vi "Config-System.vi"() -> ()   [LabVIEW 2016]
uses:
  <vilib>/Utility/error.llb/DialogType.ctl
  DAQ-Display/PanelSplitToolkit/QueueManager.llb/CreatQueue.vi
  DAQ-Display/PanelSplitToolkit/QueueManager.llb/Remove.vi
  DAQ-Display/PanelSplitToolkit/QueueManager.llb/Destroy.vi
  DAQ-Display/PanelSplitToolkit/QueueManager.llb/Valid?.vi
  DAQ-Display/PanelSplitToolkit/QueueManager.llb/Insert.vi
panel:
  in  "关注参数个数":u8=4 min=4 max=16
  in  "Caller":string caption="文件名："
  in  "手动挑点模板":path
  in  "存储路径":path
  in  "自动挑点注释":string caption="文件名："
  in  "文件存储方式":enum16{"不连续存储", "连续存储"}(ring)=enum."连续存储"
  in  "挑点模式":enum16{"不挑点", "自动挑点", "手动挑点"}(ring)=enum."自动挑点"
  in  "文件名":string caption="文件名："
  in  "默认波形图个数":u8=4 min=1 max=4
  in  "挑点间隔":i32=2
  # "存储设置"
  # "存储方式："
  # "文件夹路径："
  # "默认文件名："
  # "挑点设置"
  # "挑点模式："
  # "自动挑点间隔："
  # "秒"
  # "手动挑点模板："
  # "自动挑点注释："
  # "显示设置"
  # "个"
  # "默认图形窗口 :"
  # "个"
  # "关注参数个数 :"
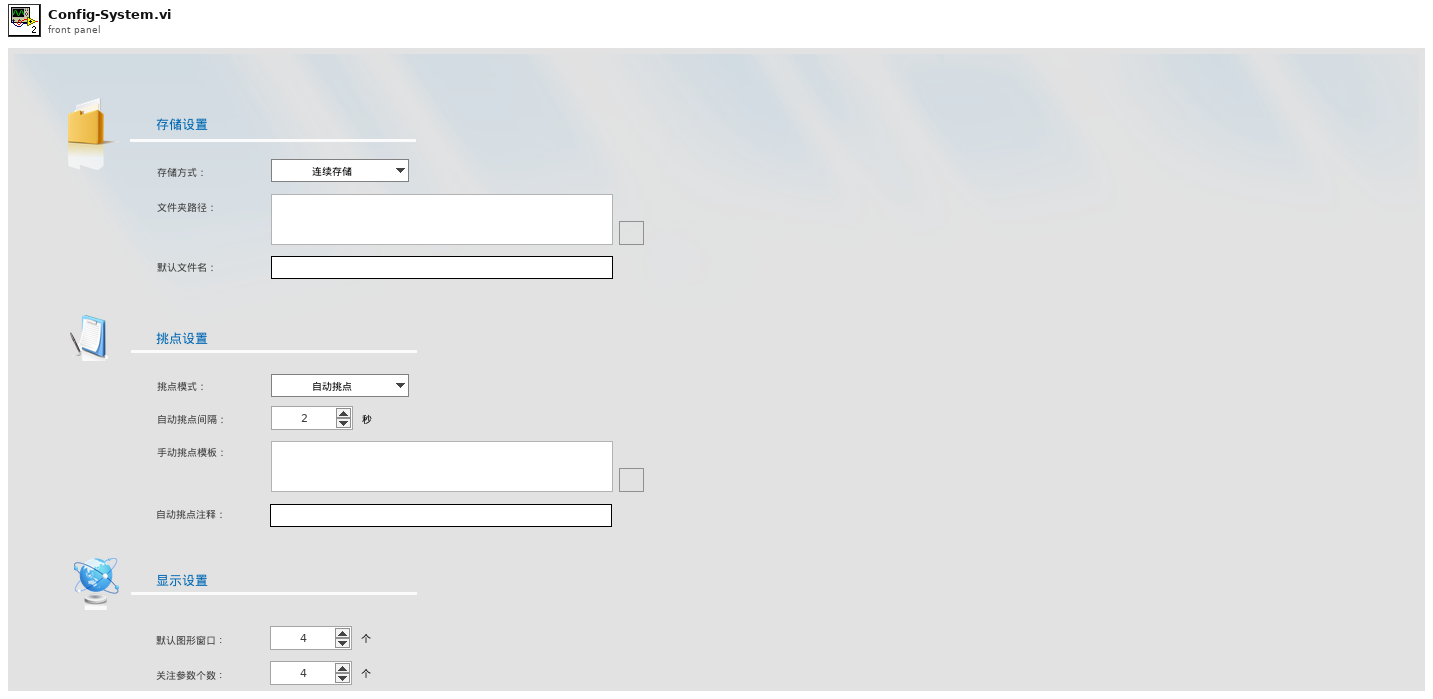
[diagram p1: front panel]
types:
  T1 = cluster{"error":errorcluster, "LocalQ":cluster{"LQName":string, "LQEvent":string, "LQData":variant}, "HighQ":cluster{"HQName":string, "HQEvent":string, "HQData":variant}}
  T2 = enum32{"Invalid", "Standard", "Closed", "Hidden", "Minimized", "Maximized"}
  T3 = typedef "DialogType.ctl" = u16
  T4 = typedef "Global para Config.ctl" = cluster{"连续存储设置":cluster{"Save Mode":i32, "Sel Save Mode":i32, "FolderPath":path, "Filename":string, "Explation":string, "AutoPoint":i32, "Template":path}, "Latest Prj":path, "Tdms Ref*":refnum<k34>, "默认波形图个数":u8, "列表列数":u8}
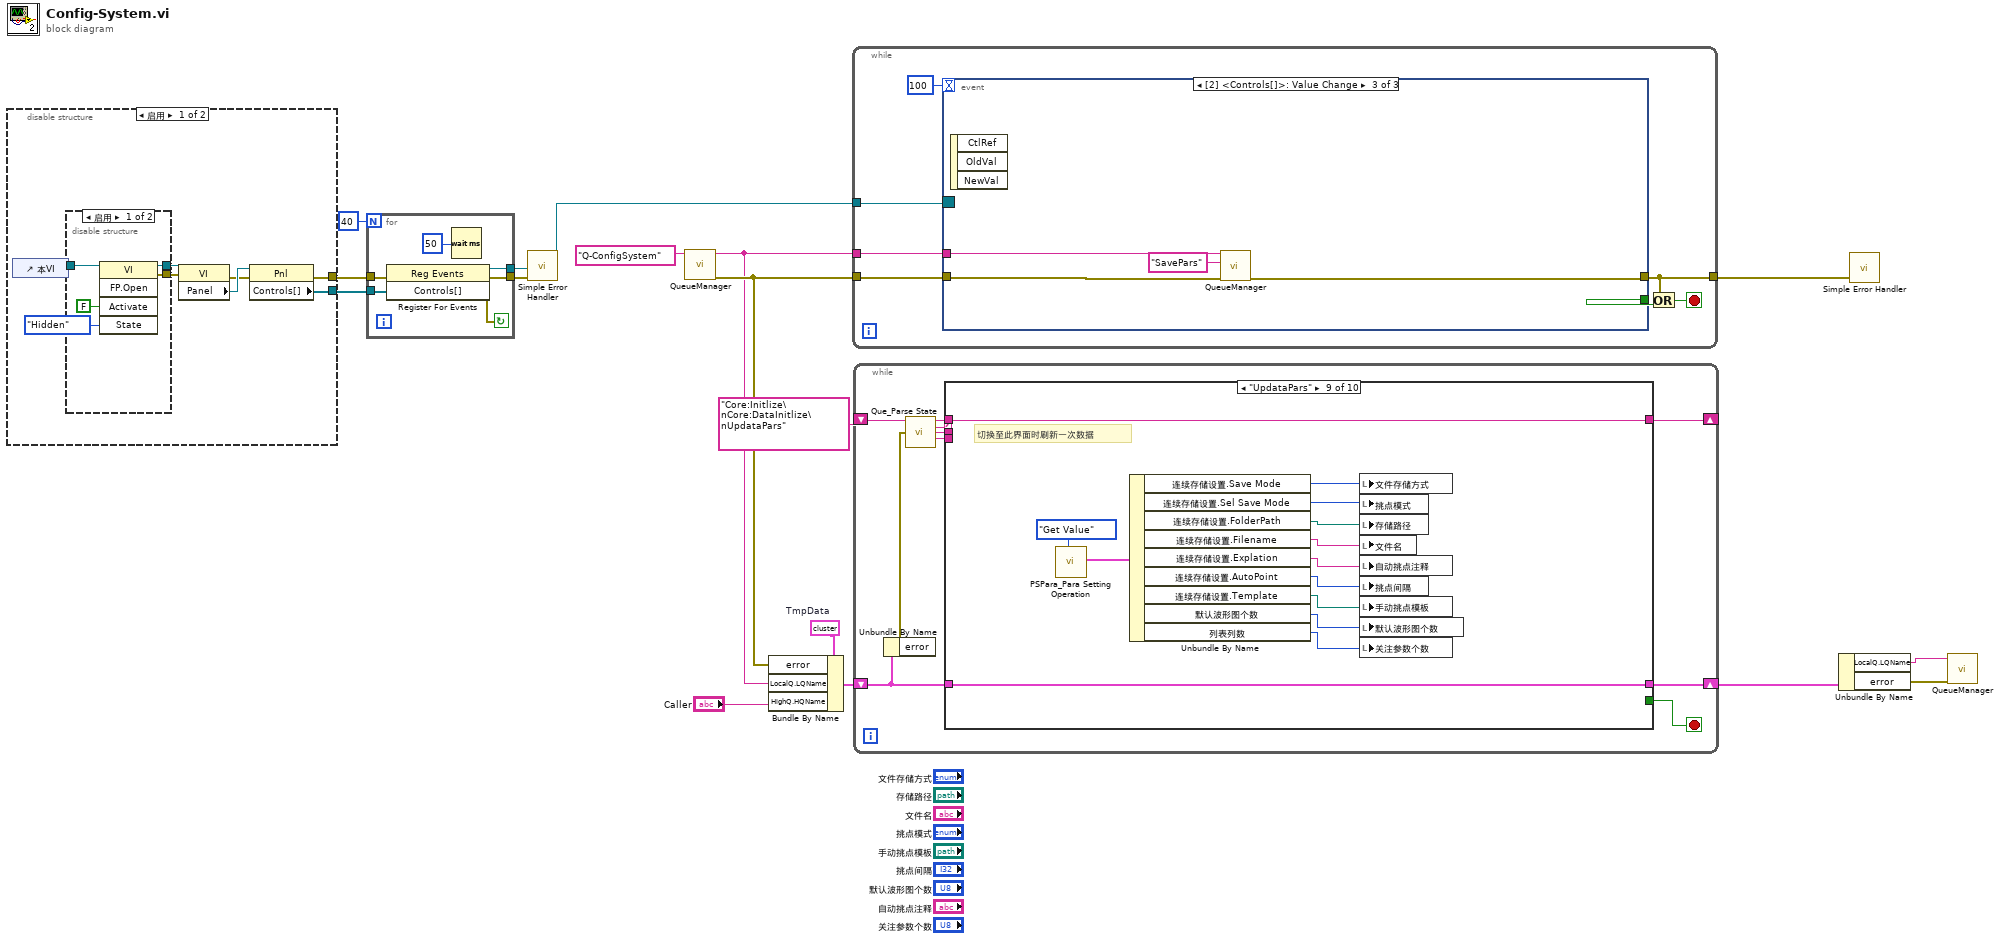
[diagram p0: block diagram]
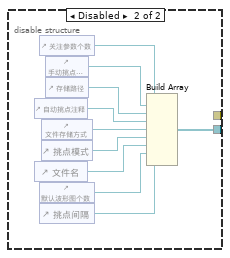
[diagram p3: hidden frame]
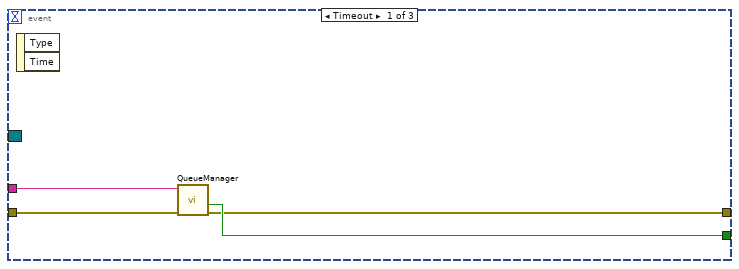
[diagram p4: hidden frame]
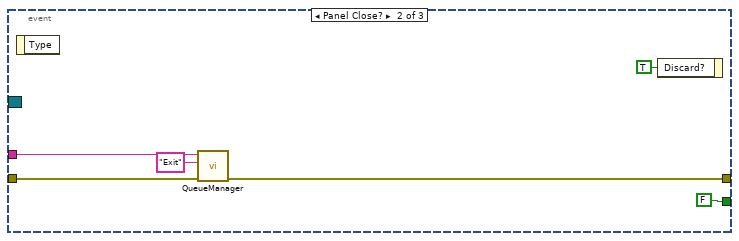
[diagram p5: hidden frame]
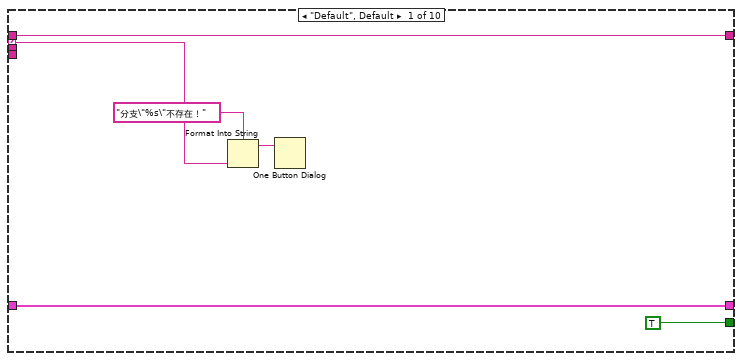
[diagram p6: hidden frame]
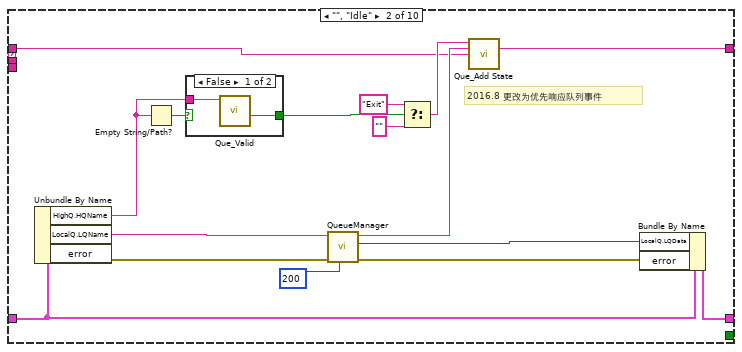
[diagram p7: hidden frame]
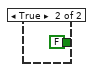
[diagram p8: hidden frame]
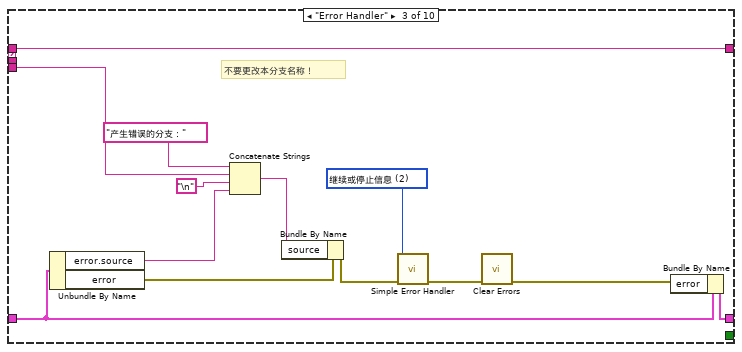
[diagram p9: hidden frame]
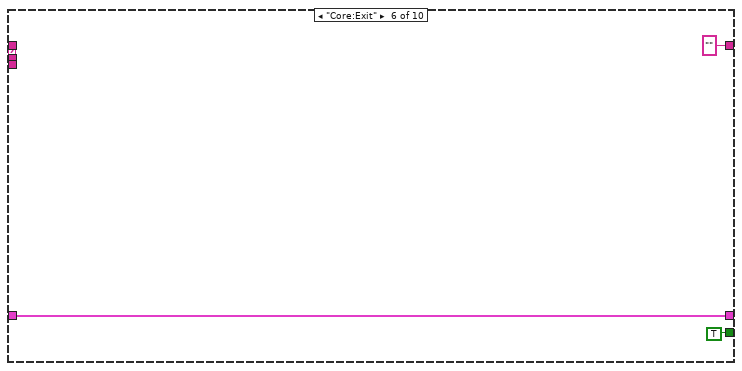
[diagram p12: hidden frame]
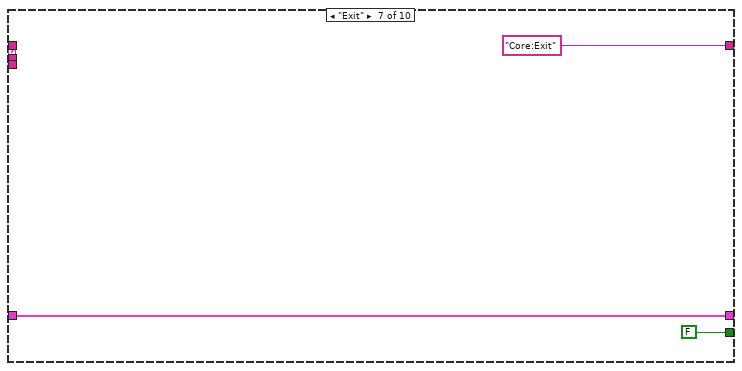
[diagram p13: hidden frame]
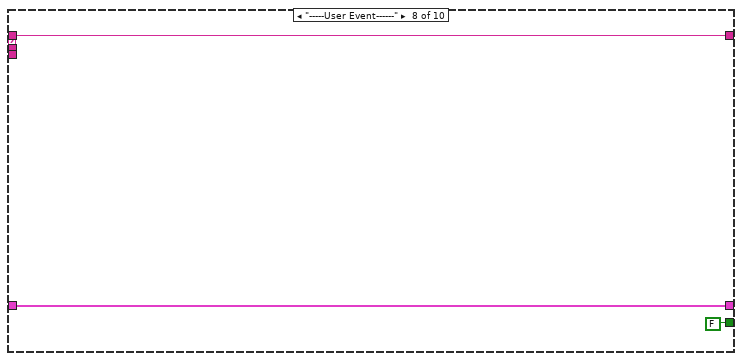
[diagram p14: hidden frame]
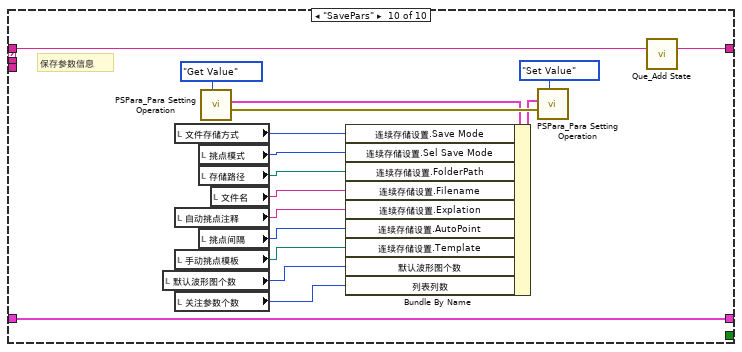
[diagram p15: hidden frame]
diagram:
  w12 = T1 {"error"={"status"=FALSE, "code"=0, "source"=""}, "LocalQ"={"LQName"="", "LQEvent"="", "LQData"=variant}, "HighQ"={"HQName"="", "HQEvent"="", "HQData"=variant}}  # TmpData
  n1 = disable-structure shown="启用" {
    disable-tunnel: [w21 w30] -> w5
    disable-tunnel: [w20 _] -> w4
    frame Enabled {
      n2 = control-ref of="本VI"() -> (w17:refnum<vi>)
      n3 = disable-structure shown="启用" {
        disable-tunnel: [w28 w29] -> w19
        disable-tunnel: [w27 _] -> w18
        disable-tunnel: w17 -> [w26 w29]
        frame Enabled {
          n4 = invoke class="VI" method="FP.Open"(reference=w26, "Activate"=FALSE ("激活？"), "State"=T2."Hidden" ("状态")) -> (reference out=w28:refnum<vi>, error out=w27:errorcluster)  [unwired: 2 in, 3 out]
        }
        frame Disabled {
        }
      }
      n5 = property class="VI"(reference=w19, error in=w18) -> (error out=w22:errorcluster, "Panel"=w23:refnum<vi>)  [unwired: 1 out]
      n6 = property class="Pnl"(reference=w23, error in=w22) -> (error out=w20:errorcluster, "Controls[]"=w21:refnum<vi>[])  [unwired: 1 out]
    }
    frame Disabled {
      n7 = control-ref of="自动挑点注释"() -> (w36:refnum<vi>)
      n8 = control-ref of="文件名"() -> (w33:refnum<vi>)
      n9 = control-ref of="关注参数个数"() -> (w39:refnum<vi>)
      n10 = control-ref of="默认波形图个数"() -> (w32:refnum<vi>)
      n11 = control-ref of="挑点间隔"() -> (w31:refnum<vi>)
      n12 = control-ref of="文件存储方式"() -> (w35:refnum<vi>)
      n13 = control-ref of="挑点模式"() -> (w34:refnum<vi>)
      n14 = control-ref of="手动挑点模板"() -> (w38:refnum<vi>)
      n15 = control-ref of="存储路径"() -> (w37:refnum<vi>)
      n16 = Build Array(w39, w38, w37, w36, w35, w34, w33, w32, w31) -> (w30:refnum<vi>[])
    }
  }
  n17 = for {
    N: 40 -> [_]
    tunnel: w5 -> [w44]
    tunnel: [w42] -> w3
    tunnel: w4 -> [w43]
    tunnel: [w40] -> w1
    stop <- w40 continue-if-true
    n18 = register-events(error in=w43, w44) -> (reference out=w42:refnum<event-registration>, error out=w40:errorcluster)  [unwired: 1 in]
    n19 = Wait (ms)(milliseconds to wait=u32 50 ("等待时间（毫秒）")) -> ()  [unwired: 1 out]
  }
  n20 = call <vilib>:"Simple Error Handler.vi"("error in (no error)"=w1) -> ()  [unwired: 4 in, 5 out]
  n21 = call-poly "QueueManager.vi"("QueueName"="Q-ConfigSystem") -> ("error out"=w8:errorcluster, "QueueName out"=w6:string)  [unwired: 9 in]
  n22 = Bundle By Name(cluster=w12, "error"=w8, "LocalQ.LQName"=w6, "HighQ.HQName"="Caller") -> (w11:T1)
  n23 = while {
    tunnel: w8 -> [w50]
    tunnel: w6 -> [w51]
    tunnel: [w47] -> w13
    tunnel: w3 -> [w45]
    stop <- w48 stop-if-true
    n24 = event shown="[2] <Controls[]>: Value Change" {
      selector: w45 -> [_ _ _]
      dyn-events: _ -> [_ _ _]
      timeout: 100 -> [_ _ _]
      tunnel: [w53 FALSE _] -> w49
      tunnel: w51 -> [w55 w60 w64]
      tunnel: w50 -> [w54 w59 w65]
      tunnel: [w52 w58 w63] -> w47
      event Timeout {
        n25 = event-data() -> ()  [unwired: 1 in, 2 out]
        n26 = call-poly "QueueManager.vi"("error in (no error)"=w54, "Queue Name(unamed)"=w55) -> ("error out"=w52:errorcluster, "Not Exist?"=w53:bool)  [unwired: 8 in]
      }
      event Panel Close? {
        n27 = event-data() -> ()  [unwired: 1 in, 1 out]
        n28 = call-poly "QueueManager.vi"("error in"=w59, "Event"="Exit", "QueueName"=w60) -> ("error out"=w58:errorcluster)  [unwired: 7 in, 1 out]
        n29 = event-data("Discard?"=TRUE ("放弃？")) -> ()  [unwired: 1 in, 1 out]
      }
      event Value Change {
        n30 = event-data() -> ()  [unwired: 1 in, 3 out]
        n31 = call-poly "QueueManager.vi"("error in"=w65, "Event"="SavePars", "QueueName"=w64) -> ("error out"=w63:errorcluster)  [unwired: 7 in, 1 out]
      }
    }
    n32 = Or(x=w47, y=w49) -> (x .or. y?=w48:bool)
  }
  n33 = while {
    shift-right: [w69] -> w14
    shift-left: w11 -> [w70]
    shift-right: [w68] -> _
    shift-left: "Core:Initlize\nCore:DataInitlize\nUpdataPars" -> [w75]
    stop <- w72 stop-if-true
    n34 = Unbundle By Name(w70) -> ("error"=w71:errorcluster)
    n35 = call "Que_Parse State.vi"("State Queue"=w75, "Error In (no error)"=w71) -> ("Remaining States"=w74:string, "Current State"=w73:string, "Arguments"=w67:string, "PreState"=w66:string)  [unwired: 10 in]
    n36 = case shown="\"UpdataPars\"" w73 {
      selector: w73 -> [w79 _ _ _ _ _ _ _ _ _]
      tunnel: w74 -> [w80 w82 w113 w115 w117 _ _ w124 w138 w155]
      tunnel: w67 -> [_ _ _ _ _ _ _ _ _ _]
      tunnel: [TRUE _ _ _ _ TRUE FALSE FALSE _ _] -> w72
      tunnel: w70 -> [w81 w92 w110 w114 w116 w119 w122 w125 w139 w156]
      tunnel: [w81 w96 w109 w114 w116 w119 w122 w125 w139 w156] -> w69
      tunnel: [w80 w94 w113 w115 w117 "" ("Remaining States") "Core:Exit" ("Remaining States") w124 w138 w154] -> w68
      tunnel: w66 -> [_ _ w107 _ _ _ _ _ _ _]
      frame "Default", Default {
        n37 = Format Into String(format string="分支\"%s\"不存在！" ("格式字符串"), w79) -> (resulting string=w78:string)  [unwired: 2 in, 1 out]
        n38 = One Button Dialog(message=w78) -> ()  [unwired: 1 in, 1 out]
      }
      frame "", "Idle" {
        # "2016.8 更改为优先响应队列事件"
        n39 = Unbundle By Name(w92) -> ("HighQ.HQName"=w86:string, "LocalQ.LQName"=w91:string, "error"=w90:errorcluster)
        n40 = Empty String/Path?(string/path=w86) -> (empty?=w89:bool)
        n41 = case shown="False" w89 {
          tunnel: [w99 FALSE ("Not Exist?")] -> w88
          tunnel: w86 -> [w98 _]
          frame False {
            n42 = call "Que_Valid.vi"("Queue Name(unamed)"=w98) -> ("Not Exist?"=w99:bool)  [unwired: 9 in, 1 out]
          }
          frame True {
          }
        }
        n43 = call-poly "QueueManager.vi"("Time out(-1)"=200, "error in (no error)"=w90, "Queue Name"=w91) -> ("error out"=w97:errorcluster, "Data"=w95:variant, "Event"=w83:string)  [unwired: 5 in, 1 out]
        n44 = Select(t="Exit" ("Event"), s=w88, f="") -> (s? t:f=w84:string)
        n45 = call "Que_Add State.vi"("State(s) in Front (\"\")"=w84, "State(s) in (\"\")"=w83, "State(s) at Back (\"\")"=w82) -> ("States Out"=w94:string)  [unwired: 12 in]
        n46 = Bundle By Name(cluster=w92, "LocalQ.LQData"=w95, "error"=w97) -> (w96:T1)
      }
      frame "Error Handler" {
        w108 = T3 2 items=["无对话框", "确定信息", "继续或停止信息", "确定信息＋警告", "继续/停止+警告"] ("type of dialog (OK msg:1)")
        # "不要更改本分支名称！"
        n47 = Unbundle By Name(w110) -> ("error.source"=w101:string, "error"=w103:errorcluster)
        n48 = Concatenate Strings("产生错误的分支：" ("字符串"), w107, "\n", w101) -> (w104:string)
        n49 = Bundle By Name(cluster=w103, "source"=w104) -> (w102:errorcluster)
        n50 = call <vilib>:"Simple Error Handler.vi"("type of dialog (OK msg:1)"=w108, "error in (no error)"=w102) -> ("error out"=w111:errorcluster)  [unwired: 3 in, 4 out]
        n51 = call <vilib>:"Clear Errors.vi"("error in (no error)"=w111) -> ("error out"=w112:errorcluster)  [unwired: 5 in, 1 out]
        n52 = Bundle By Name(cluster=w110, "error"=w112) -> (w109:T1)
      }
      frame "Core:Initlize" {
      }
      frame "Core:DataInitlize" {
      }
      frame "Core:Exit" {
      }
      frame "Exit" {
      }
      frame "-----User Event------" {
      }
      frame "UpdataPars" {
        # "切换至此界面时刷新一次数据"
        n53 = call "PSPara_Para Setting Operation.vi"("Operation"=enum16{"Set Value", "Get Value", "Initialize"}."Get Value") -> ("_Para"=w136:T4)  [unwired: 9 in, 1 out]
        n54 = Unbundle By Name(w136) -> ("连续存储设置.Save Mode"=w135:i32, "连续存储设置.Sel Save Mode"=w134:i32, "连续存储设置.FolderPath"=w133:path, "连续存储设置.Filename"=w132:string, "连续存储设置.Explation"=w131:string, "连续存储设置.AutoPoint"=w130:i32, "连续存储设置.Template"=w129:path, "默认波形图个数"=w128:u8, "列表列数"=w127:u8)
        n55 = local write "文件存储方式"(w135) -> ()
        n56 = local write "挑点模式"(w134) -> ()
        n57 = local write "存储路径"(w133) -> ()
        n58 = local write "文件名"(w132) -> ()
        n59 = local write "自动挑点注释"(w131) -> ()
        n60 = local write "挑点间隔"(w130) -> ()
        n61 = local write "手动挑点模板"(w129) -> ()
        n62 = local write "默认波形图个数"(w128) -> ()
        n63 = local write "关注参数个数"(w127) -> ()
      }
      frame "SavePars" {
        # "保存参数信息"
        n64 = local read "默认波形图个数"() -> (w141:u8)
        n65 = local read "文件存储方式"() -> (w148:enum16{"不连续存储", "连续存储"})
        n66 = local read "自动挑点注释"() -> (w144:string)
        n67 = local read "手动挑点模板"() -> (w142:path)
        n68 = local read "关注参数个数"() -> (w140:u8)
        n69 = local read "挑点模式"() -> (w147:enum16{"不挑点", "自动挑点", "手动挑点"})
        n70 = local read "存储路径"() -> (w146:path)
        n71 = local read "挑点间隔"() -> (w143:i32)
        n72 = call "PSPara_Para Setting Operation.vi"("Operation"=enum16{"Set Value", "Get Value", "Initialize"}."Get Value") -> ("error out"=w151:errorcluster, "_Para"=w150:T4)  [unwired: 9 in]
        n73 = local read "文件名"() -> (w145:string)
        n74 = Bundle By Name(cluster=w150, "连续存储设置.Save Mode"=w148, "连续存储设置.Sel Save Mode"=w147, "连续存储设置.FolderPath"=w146, "连续存储设置.Filename"=w145, "连续存储设置.Explation"=w144, "连续存储设置.AutoPoint"=w143, "连续存储设置.Template"=w142, "默认波形图个数"=w141, "列表列数"=w140) -> (w149:T4)
        n75 = call "PSPara_Para Setting Operation.vi"("Operation"=enum16{"Set Value", "Get Value", "Initialize"}."Set Value", "error in (no error)"=w151, "_Para"=w149) -> ()  [unwired: 7 in, 2 out]
        n76 = call "Que_Add State.vi"("State(s) in (\"\")"=w155) -> ("States Out"=w154:string)  [unwired: 14 in]
      }
    }
  }
  n77 = Unbundle By Name(w14) -> ("LocalQ.LQName"=w9:string, "error"=w15:errorcluster)
  n78 = call <vilib>:"Simple Error Handler.vi"("error in (no error)"=w13) -> ()  [unwired: 4 in, 5 out]
  n79 = call-poly "QueueManager.vi"("error in (no error)"=w15, "QueeuName"=w9) -> ()  [unwired: 9 in, 1 out]
